vi "OPO_Main.vi"(8 "error in (no error)":errorcluster, 11 "port":u16=6000) -> (0 "error out":errorcluster)   [LabVIEW 2020]
panel:
  out "OPO Energy":dbl
  out "OPO wavelength":i32
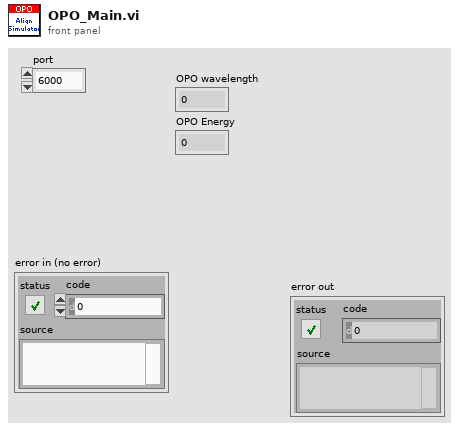
[diagram p1: front panel]
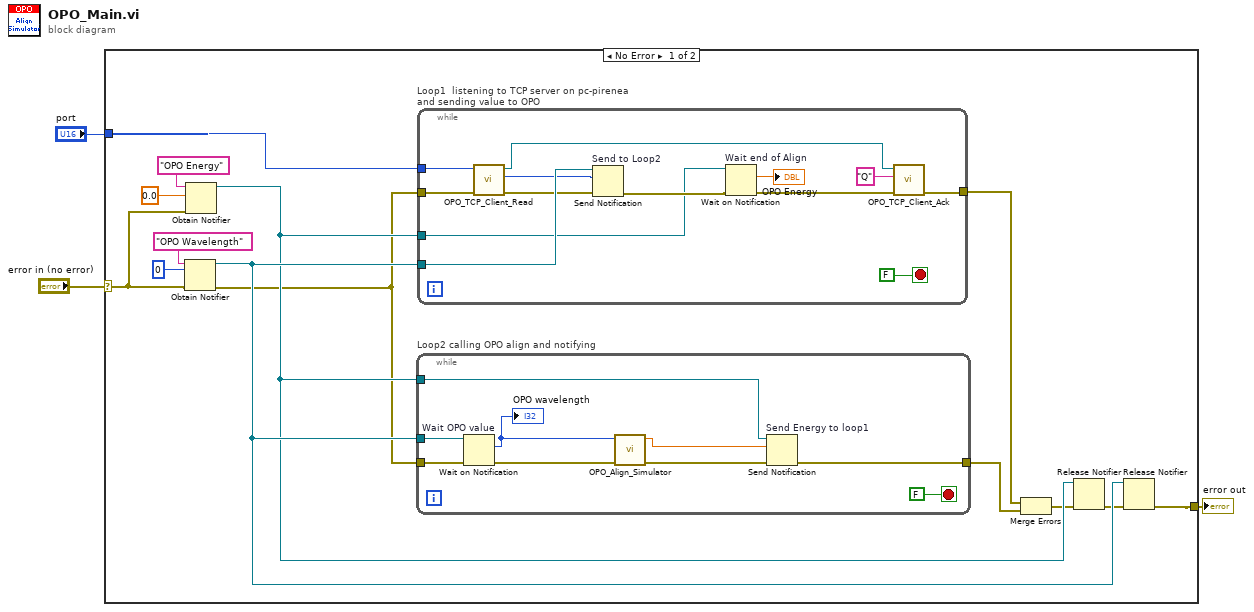
[diagram p0: block diagram]
diagram:
  n1 = case shown="No Error" "error in (no error)" {
    selector: "error in (no error)" -> [w5 w40]
    tunnel: [w16 w40] -> w2
    tunnel: "port" -> [w17 _]
    frame No Error {
      n2 = Obtain Notifier(name (unnamed)="OPO Wavelength", notification data type=0, error in (no error)=w5) -> (notifier out=w14:refnum<notifier>, error out=w4:errorcluster)  [unwired: 1 in, 1 out]
      n3 = Obtain Notifier(name (unnamed)="OPO Energy", notification data type=0.0, error in (no error)=w5) -> (notifier out=w9:refnum<notifier>)  [unwired: 1 in, 2 out]
      n4 = while "Loop2 calling OPO align and notifying" {
        tunnel: w14 -> [w26]
        tunnel: w9 -> [w23]
        tunnel: w4 -> [w25]
        tunnel: [w22] -> w15
        stop <- FALSE stop-if-true
        n5 = Wait on Notification "Wait OPO value"(notifier=w26, error in (no error)=w25) -> (notification=w19:i32, error out=w24:errorcluster)  [unwired: 2 in, 2 out]
        "OPO wavelength" <- w19
        n6 = call "OPO_Align_Simulator.vi"("error in (no error)"=w24, "OPO wavelength"=w19) -> ("error out"=w20:errorcluster, "OPO Energy"=w18:dbl)  [unwired: 8 in]
        n7 = Send Notification "Send Energy to loop1"(notification=w18, notifier=w23, error in (no error)=w20) -> (error out=w22:errorcluster)  [unwired: 1 out]
      }
      n8 = while "Loop1  listening to TCP server on pc-pirenea and sending value to OPO" {
        tunnel: w17 -> [w31]
        tunnel: w14 -> [w39]
        tunnel: w9 -> [w35]
        tunnel: [w28] -> w7
        tunnel: w4 -> [w33]
        stop <- FALSE stop-if-true
        n9 = call "OPO_TCP_Client_Read.vi"("error in (no error)"=w33, "port"=w31) -> ("error out"=w32:errorcluster, "value read"=w30:i32, "TCP Network Connection out"=w29:refnum<k5>)  [unwired: 7 in]
        n10 = Send Notification "Send to Loop2"(notification=w30, notifier=w39, error in (no error)=w32) -> (error out=w38:errorcluster)  [unwired: 1 out]
        n11 = Wait on Notification "Wait end of Align"(notifier=w35, error in (no error)=w38) -> (notification=→"OPO Energy":dbl, error out=w37:errorcluster)  [unwired: 2 in, 2 out]
        n12 = call "OPO_TCP_Client_Ack.vi"("error in (no error)"=w37, "ACK letter"="Q", "TCP Network Connection in"=w29) -> ("error out"=w28:errorcluster)  [unwired: 7 in, 1 out]
      }
      n13 = Merge Errors(w7, w15) -> (w6:errorcluster)
      n14 = Release Notifier(notifier=w9, error in (no error)=w6) -> (error out=w8:errorcluster)  [unwired: 1 in, 2 out]
      n15 = Release Notifier(notifier=w14, error in (no error)=w8) -> (error out=w16:errorcluster)  [unwired: 1 in, 2 out]
    }
    frame Error {
    }
  }
  "error out" <- w2
